vi "set cause.vi"(10 "cause":T1 {"code" format="%.0x"}, 11 "exception in":T1 {"code" format="%.0x"}) -> (3 "exception out":T1 {"code" format="%.0x"})   [LabVIEW 2013, in "exception.lvlib"]
uses:
  exception.lvlib
  exception.ctl
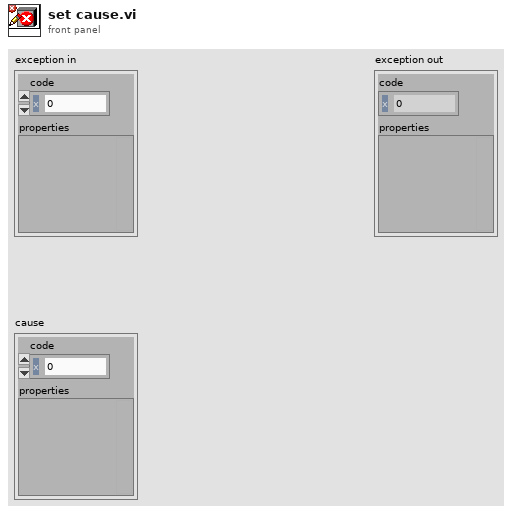
[diagram p1: front panel]
types:
  T1 = typedef "exception.lvlib/exception.ctl" = cluster{"code":i32, "properties":variant}
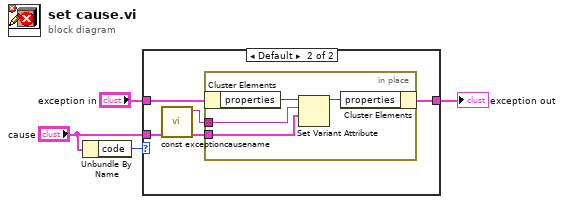
[diagram p0: block diagram]
diagram:
  n1 = Unbundle By Name("cause") -> ("code"=w1:i32)
  n2 = case shown="Default" w1 {
    tunnel: "exception in" -> [w5 w9]
    tunnel: [w5 w8] -> w3
    tunnel: "cause" -> [_ w6]
    frame 0 {
    }
    frame Default {
      n3 = call "const exceptioncausename.vi"() -> ("label"=w7:string)  [unwired: 11 in]
      n4 = in-place {
        in-place-border: w7 -> [w11]
        in-place-border: w6 -> [w10]
        n5 = in-place-cluster #1(w9) -> ("properties"=w13:variant)
        n6 = Set Variant Attribute(Variant=w13, name=w11, value=w10) -> (Variant out=w12:variant)  [unwired: 1 in, 2 out]
        n7 = in-place-cluster #1("properties"=w12) -> (w8:T1)
      }
    }
  }
  "exception out" <- w3
